vi "Testing_Original.vi"() -> ()   [LabVIEW 2021]
uses:
  Motion_Panel_State_Machine/Motion_Panel_State_Machine.lvclass
  C:/Program Files (x86)/Hyper State Machine Framework/SSW_Panel_Adaptive.lvlibp/Panel_Adaptive/Panel_Adaptive.lvclass
  C:/Program Files (x86)/Hyper State Machine Framework/SSW_Hyper_State_Machine.lvlibp/State_Machine_Class/Main_State_Machine/Hyper_State_Machine.lvclass
  DIO_Panel_State_Machine/DIO_Panel_State_Machine.lvclass
  Class 1/Panel1.lvclass
  C:/Program Files (x86)/Hyper State Machine Framework/SSW_Panel_Adaptive.lvlibp/Panel_Interface/Panel_Interface.lvclass
  Class 3/Panel3.lvclass
  Class 2/Panel2.lvclass
  C:/Program Files (x86)/Hyper State Machine Framework/SSW_Hyper_State_Machine.lvlibp/State_Machine_Class/State_Machine_Module.llb/Lock_Unlock.ctl
  C:/Program Files (x86)/Hyper State Machine Framework/SSW_Hyper_State_Machine.lvlibp/State_Machine_Class/State_Machine_Module.llb/State Machine.ctl
  C:/Program Files (x86)/Hyper State Machine Framework/SSW_Hyper_State_Machine.lvlibp
panel:
  out "Block_Chain":refnum<class "Hyper_State_Machine.lvclass">[](array[class])
  out "Commander":refnum<class "Hyper_State_Machine.lvclass">
  out "Exit":bool
  out "HPSMO4-20":refnum<class "Panel_Adaptive.lvclass">[](array[class])
  out "HPSMO2":refnum<class "Panel_Adaptive.lvclass">
  out "HSMO4-20":refnum<class "Hyper_State_Machine.lvclass">[](array[class])
  out "HSMO3":refnum<class "Hyper_State_Machine.lvclass">
  out "HPSMO3":refnum<class "DIO_Panel_State_Machine.lvclass">
  out "HSMO2":refnum<class "Hyper_State_Machine.lvclass">
  out "HSMO1":refnum<class "Hyper_State_Machine.lvclass">
  out "HPSMO1":refnum<class "Motion_Panel_State_Machine.lvclass">
  in  "Reset_State":bool
  in  "Reset_All":bool
  in  "Change_VI_All":bool
  in  "Panel Index":i32=1 min=1 max=20
  in  "Implementation":u16(ring)
  in  "Change_VI":bool
  out "Main_Active":bool
  in  "Main_Interval(s)":dbl=0.025 format="%.0p"
  in  "Option Button":bool=TRUE
  in  "Time Target (s)":dbl=30.0 format="%#_13g"
  in  "lock All":bool
  in  "Unlock":bool
  out "All_Values":variant[][](array[variant])
  out "error out":errorcluster
  in  "Exit":bool
  in  "Tab Control":T1(tab)
  in  "Swap3-4":bool
  in  "Swap1-4":bool
  in  "Swap2-3":bool
  in  "Swap1-2":bool
  out "Active 3":bool
  out "Active 2":bool
  out "Timing 3":dbl
  out "Timing 2":dbl
  out "Active 1":bool
  out "Timing 1":dbl
  out "Timing 20":dbl
  out "Active 20":bool
  out "Get_Current State_Sub Panel_1":string
  out "HSMO1_ID":u32 format="%08x"
  out "HSMO1 Running":bool
  in  "Request_Release":bool
  out "Command_Lock":bool
  out "Commander_State":string
  out "HSMO_Commander_ID":u32 format="%08x"
  out "Block Chain Message":string
  # "Local"
  # "Panel Method"
  # "State Method"
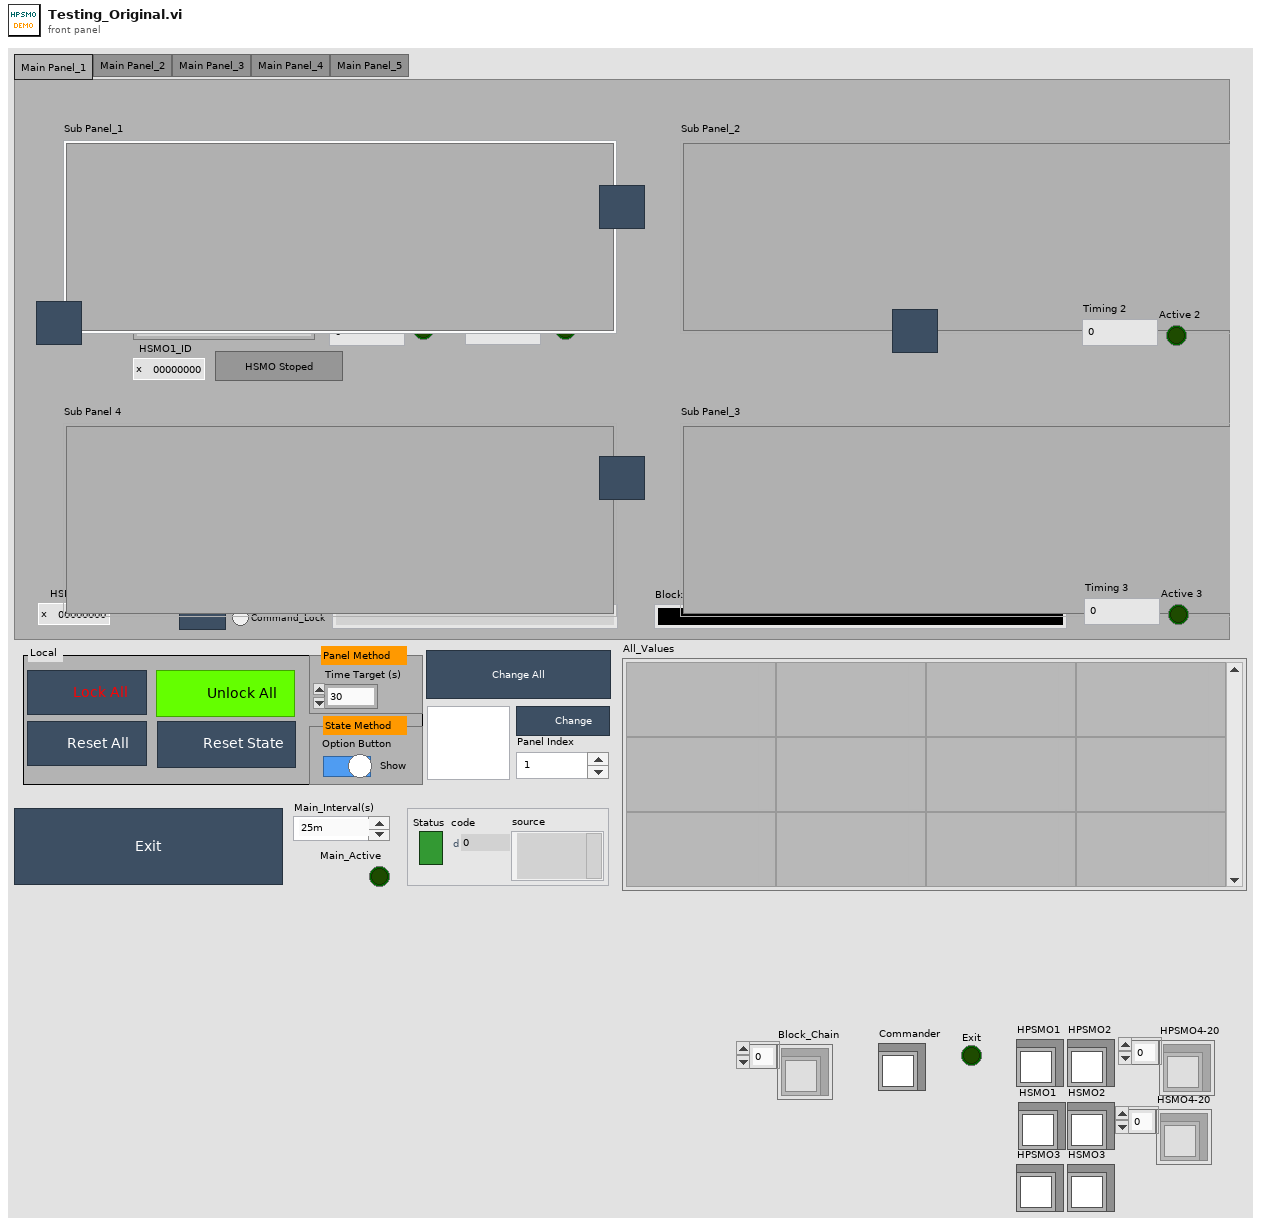
[diagram p1: front panel]
types:
  T1 = enum32{"Main Panel_1", "Main Panel_2", "Main Panel_3", "Main Panel_4", "Main Panel_5"}
  T2 = typedef "SSW_Hyper_State_Machine.lvlibp/State Machine.ctl" = cluster{"Command":string, "Data":variant}
  T3 = typedef "SSW_Hyper_State_Machine.lvlibp/Lock_Unlock.ctl" = cluster{"Action_Mode (Get)":enum16{"Set", "Get"}, "Action_Set (False)":bool, "State_In (Wait)":string}
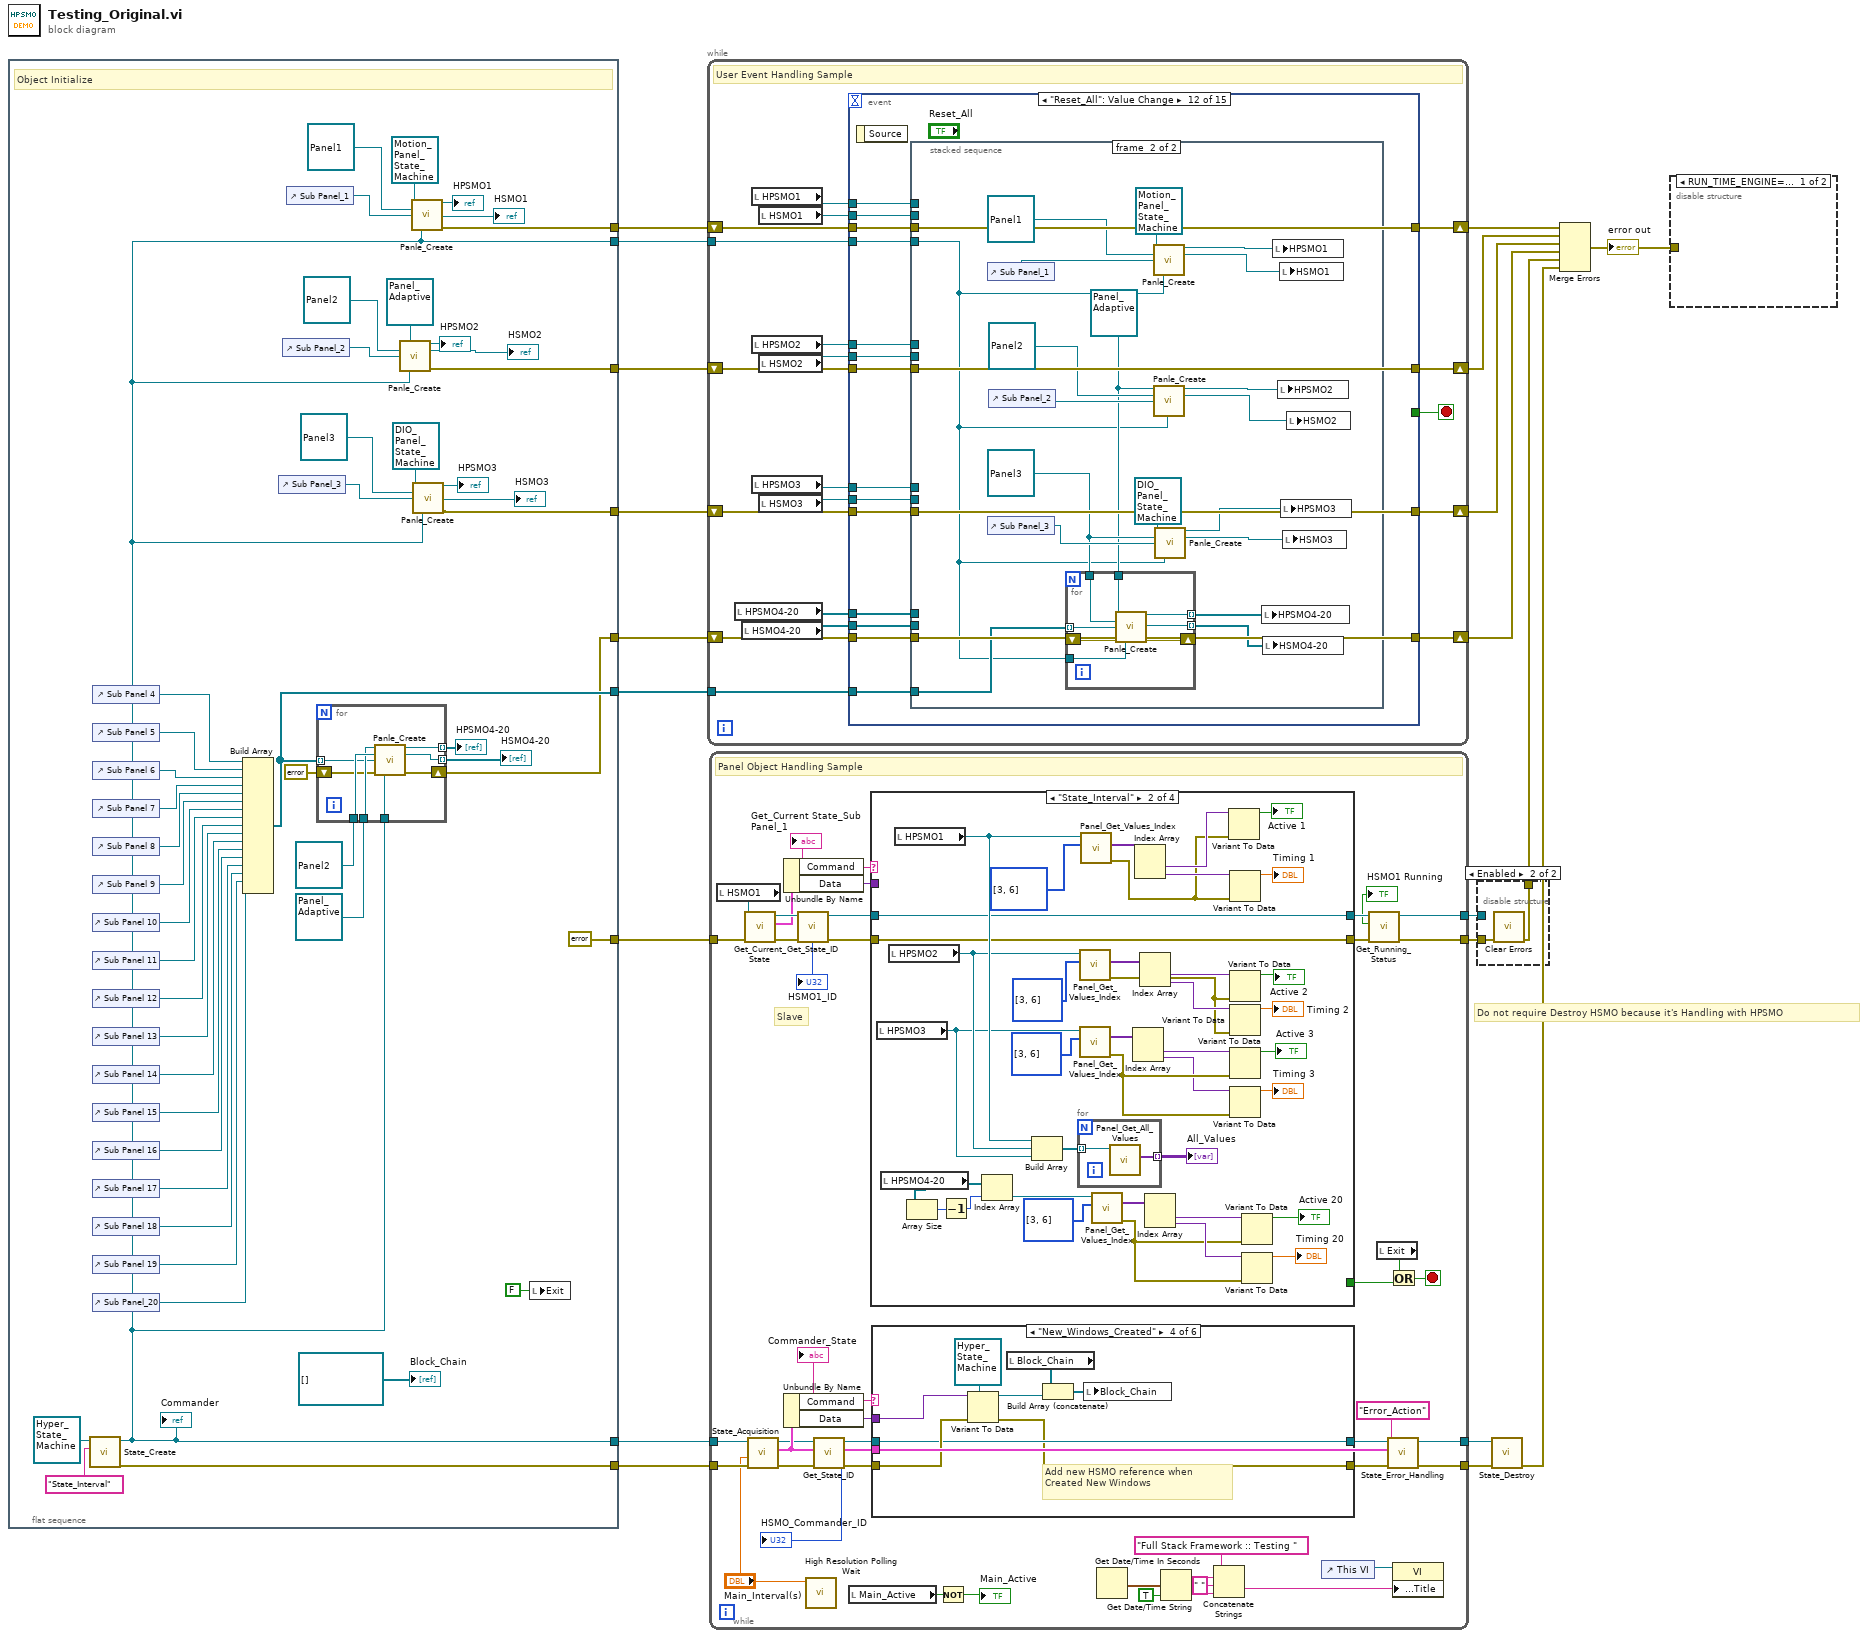
[diagram p0: block diagram]
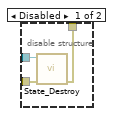
[diagram p2: hidden frame]
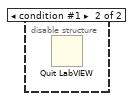
[diagram p3: hidden frame]
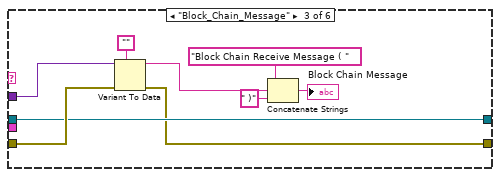
[diagram p6: hidden frame]
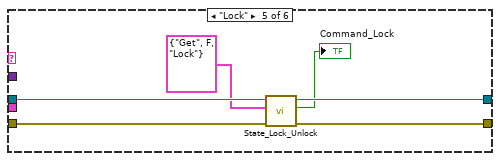
[diagram p7: hidden frame]
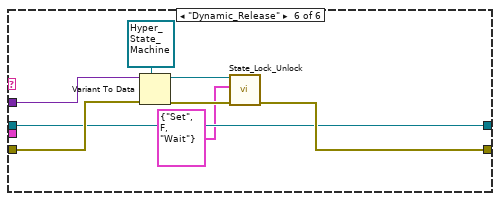
[diagram p8: hidden frame]
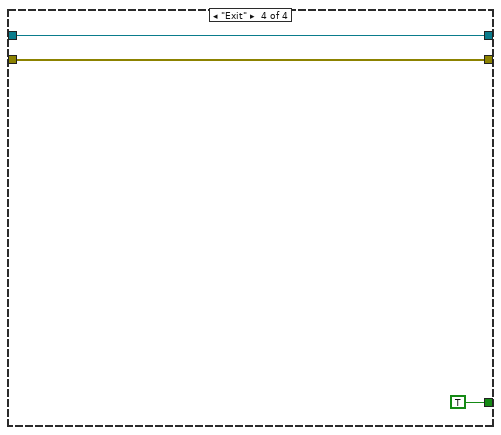
[diagram p11: hidden frame]
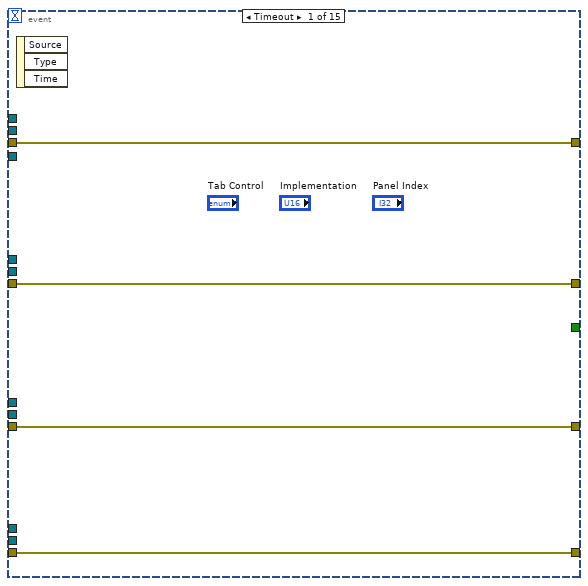
[diagram p12: hidden frame]
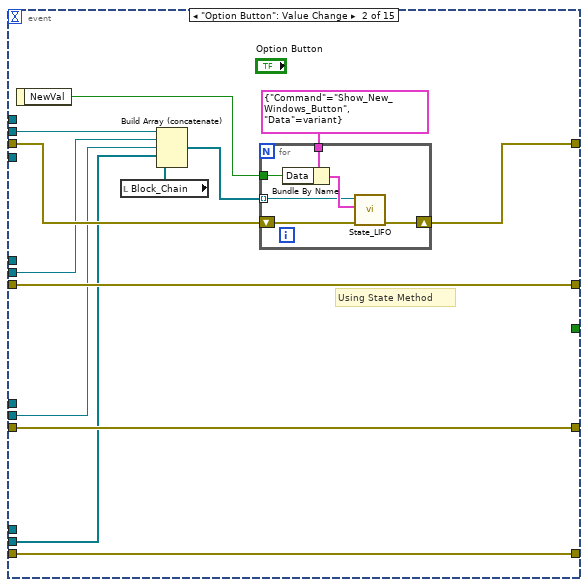
[diagram p13: hidden frame]
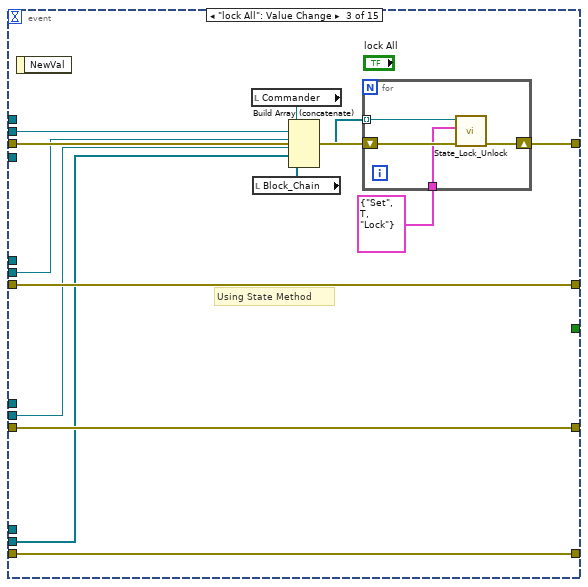
[diagram p14: hidden frame]
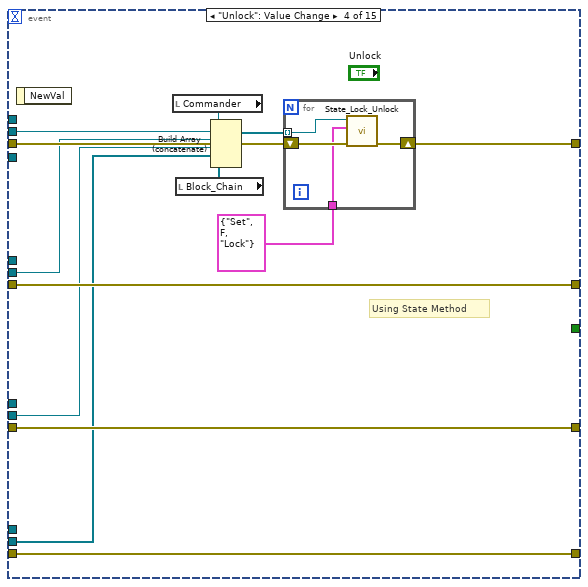
[diagram p15: hidden frame]
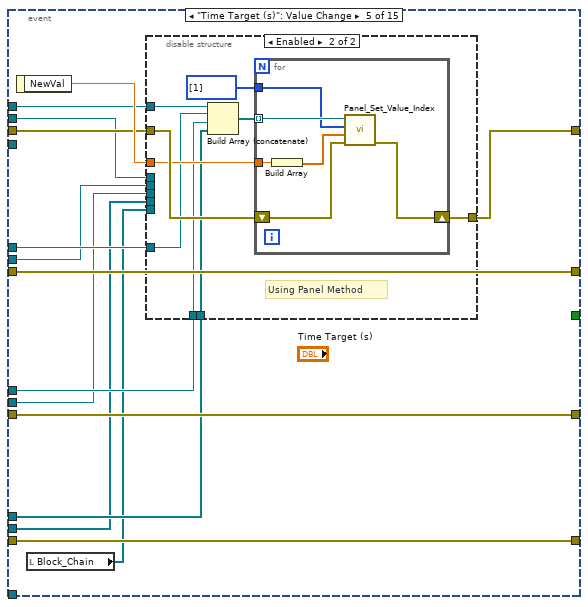
[diagram p16: hidden frame]
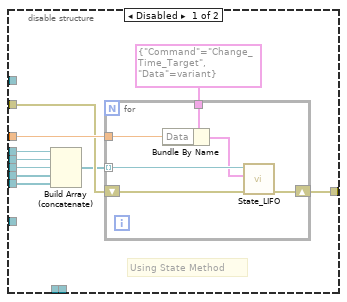
[diagram p17: hidden frame]
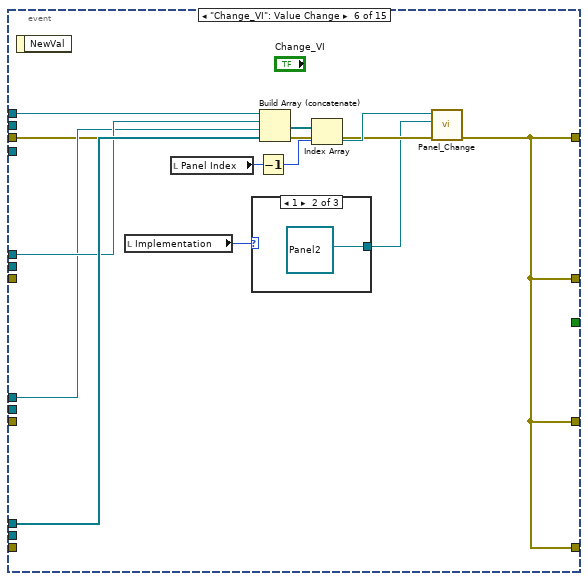
[diagram p18: hidden frame]
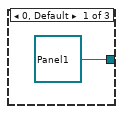
[diagram p19: hidden frame]
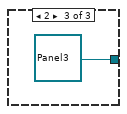
[diagram p20: hidden frame]
diagram:
  # "Do not require Destroy HSMO because it's Handling with HPSMO"
  n1 = flat-sequence {
    tunnel: [w41] -> w15
    tunnel: [w39] -> w9
    tunnel: [w38] -> w14
    tunnel: [w37] -> w13
    tunnel: [w32] -> w12
    tunnel: [errorcluster {"status"=FALSE, "code"=0, "source"=""} ("error in (no error)")] -> w4
    tunnel: [w21] -> w3
    tunnel: [w23] -> w2
    tunnel: [w21] -> w1
    frame #0 {
      # "Object Initialize"
      n2 = call-dynamic "State_Create.vi"("State_Interval_Name"="State_Interval", "State_Machine_Class in"=refnum<class "Hyper_State_Machine.lvclass"> refnum) -> ("error out"=w23:errorcluster, "State_Machine_Class out"=w21:refnum<class "Hyper_State_Machine.lvclass">)  [unwired: 7 in, 1 out]
      "Commander" <- w21
      n3 = control-ref of="Sub Panel 4"() -> (w64:refnum<vi>)
      n4 = control-ref of="Sub Panel 5"() -> (w63:refnum<vi>)
      n5 = control-ref of="Sub Panel 6"() -> (w62:refnum<vi>)
      n6 = control-ref of="Sub Panel 7"() -> (w61:refnum<vi>)
      n7 = control-ref of="Sub Panel 8"() -> (w60:refnum<vi>)
      n8 = control-ref of="Sub Panel 9"() -> (w59:refnum<vi>)
      n9 = control-ref of="Sub Panel 10"() -> (w58:refnum<vi>)
      n10 = control-ref of="Sub Panel 11"() -> (w57:refnum<vi>)
      n11 = control-ref of="Sub Panel 12"() -> (w56:refnum<vi>)
      n12 = control-ref of="Sub Panel 13"() -> (w55:refnum<vi>)
      n13 = control-ref of="Sub Panel 14"() -> (w54:refnum<vi>)
      n14 = control-ref of="Sub Panel 15"() -> (w53:refnum<vi>)
      n15 = control-ref of="Sub Panel 16"() -> (w52:refnum<vi>)
      n16 = control-ref of="Sub Panel 17"() -> (w51:refnum<vi>)
      n17 = control-ref of="Sub Panel 18"() -> (w50:refnum<vi>)
      n18 = control-ref of="Sub Panel 19"() -> (w49:refnum<vi>)
      n19 = control-ref of="Sub Panel_20"() -> (w47:refnum<vi>)
      n20 = Build Array(w64, w63, w62, w61, w60, w59, w58, w57, w56, w55, w54, w53, w52, w51, w50, w49, w47) -> (w41:refnum<vi>[])
      n21 = control-ref of="Sub Panel_3"() -> (w46:refnum<vi>)
      n22 = control-ref of="Sub Panel_2"() -> (w28:refnum<vi>)
      n23 = control-ref of="Sub Panel_1"() -> (w45:refnum<vi>)
      n24 = for {
        shift-right: [w73] -> w38
        shift-left: errorcluster {"status"=FALSE, "code"=0, "source"=""} ("error out") -> [w75]
        tunnel: w41 -> [w74] mode=indexing
        tunnel: [w72] -> w48 mode=indexing
        tunnel: refnum<class "Panel2.lvclass"> refnum ("Class 2.lvclass") -> [w77]
        tunnel: refnum<class "Panel_Adaptive.lvclass"> refnum ("SSW_Panel_Adaptive.lvlibp:Panel_Adaptive.lvclass") -> [w76]
        tunnel: [w71] -> w30 mode=indexing
        tunnel: w21 -> [w70]
        n25 = call-dynamic "Panle_Create.vi"("Hyper_Panel_State_Machine in"=w76, "Panel_Source"=w77, "Panel_Ref"=w74, "error in (no error)"=w75, "Parent_State"=w70) -> ("Hyper_Panel_State_Machine out"=w71:refnum<class "Panel_Adaptive.lvclass">, "This_State"=w72:refnum<class "Hyper_State_Machine.lvclass">, "error out"=w73:errorcluster)  [unwired: 8 in]
      }
      "HSMO4-20" <- w48
      "HPSMO4-20" <- w30
      n26 = call-dynamic "Panle_Create.vi"("Hyper_Panel_State_Machine in"=refnum<class "Panel_Adaptive.lvclass"> refnum ("SSW_Panel_Adaptive.lvlibp:Panel_Adaptive.lvclass"), "Panel_Source"=refnum<class "Panel2.lvclass"> refnum ("Class 2.lvclass"), "Panel_Ref"=w28, "Parent_State"=w21) -> ("Hyper_Panel_State_Machine out"=→"HPSMO2":refnum<class "Panel_Adaptive.lvclass">, "This_State"=→"HSMO2":refnum<class "Hyper_State_Machine.lvclass">, "error out"=w32:errorcluster)  [unwired: 9 in]
      n27 = call-dynamic "Panle_Create.vi"("Hyper_Panel_State_Machine in"=refnum<class "Motion_Panel_State_Machine.lvclass"> refnum ("Motion_Panel_State_Machine.lvclass"), "Panel_Source"=refnum<class "Panel1.lvclass"> refnum ("Class 1.lvclass"), "Panel_Ref"=w45, "Parent_State"=w21) -> ("Hyper_Panel_State_Machine out"=→"HPSMO1":refnum<class "Motion_Panel_State_Machine.lvclass">, "This_State"=→"HSMO1":refnum<class "Hyper_State_Machine.lvclass">, "error out"=w39:errorcluster)  [unwired: 9 in]
      n28 = call-dynamic "Panle_Create.vi"("Hyper_Panel_State_Machine in"=refnum<class "DIO_Panel_State_Machine.lvclass"> refnum ("DIO_Panel_State_Machine.lvclass"), "Panel_Source"=refnum<class "Panel3.lvclass"> refnum ("Class 3.lvclass"), "Panel_Ref"=w46, "Parent_State"=w21) -> ("Hyper_Panel_State_Machine out"=→"HPSMO3":refnum<class "DIO_Panel_State_Machine.lvclass">, "This_State"=→"HSMO3":refnum<class "Hyper_State_Machine.lvclass">, "error out"=w37:errorcluster)  [unwired: 9 in]
      n29 = local write "Exit"(FALSE ("Exit")) -> ()
      "Block_Chain" <- refnum<class "Hyper_State_Machine.lvclass">[] [] ("Block_Chain")
    }
  }
  n30 = while {
    tunnel: w15 -> [w91]
    shift-right: [w92] -> w16
    shift-left: w9 -> [w83]
    shift-right: [w95] -> w20
    shift-left: w12 -> [w81]
    shift-right: [w94] -> w19
    shift-left: w13 -> [w82]
    shift-right: [w93] -> w17
    shift-left: w14 -> [w80]
    tunnel: w1 -> [w78]
    stop <- w96 stop-if-true
    # "User Event Handling Sample"
    n31 = local read "HPSMO4-20"() -> (w87:refnum<class "Panel_Adaptive.lvclass">[])
    n32 = local read "HSMO4-20"() -> (w86:refnum<class "Hyper_State_Machine.lvclass">[])
    n33 = local read "HPSMO1"() -> (w90:refnum<class "Motion_Panel_State_Machine.lvclass">)
    n34 = local read "HPSMO2"() -> (w89:refnum<class "Panel_Adaptive.lvclass">)
    n35 = local read "HPSMO3"() -> (w85:refnum<class "DIO_Panel_State_Machine.lvclass">)
    n36 = local read "HSMO1"() -> (w79:refnum<class "Hyper_State_Machine.lvclass">)
    n37 = local read "HSMO2"() -> (w88:refnum<class "Hyper_State_Machine.lvclass">)
    n38 = local read "HSMO3"() -> (w84:refnum<class "Hyper_State_Machine.lvclass">)
    n39 = event shown="[11] \"Reset_All\": Value Change" {
      selector: _ -> [_ _ _ _ _ _ _ _ _ _ _ _ _ _ _]
      dyn-events: _ -> [_ _ _ _ _ _ _ _ _ _ _ _ _ _ _]
      timeout: _ -> [_ _ _ _ _ _ _ _ _ _ _ _ _ _ _]
      tunnel: [_ _ _ _ _ _ _ _ _ _ _ _ _ _ w365] -> w96
      tunnel: w83 -> [w98 w113 w131 w148 w166 w201 _ w240 w245 w261 w269 w281 w337 w350 w364]
      tunnel: [_ w112 w132 w149 w168 w209 w223 w239 w245 w258 w269 w281 w337 w347 w362] -> w92
      tunnel: w90 -> [_ _ _ _ w159 w204 w219 w233 _ w254 _ w282 _ _ w356]
      tunnel: w79 -> [_ w105 w125 w140 w158 _ _ _ _ _ _ w286 w333 w349 w352]
      tunnel: w88 -> [_ w104 w124 w141 w157 _ _ _ _ _ _ w285 w332 _ _]
      tunnel: w84 -> [_ w103 w123 w138 w156 _ _ _ _ _ _ w284 w331 _ _]
      tunnel: w89 -> [_ _ _ _ w160 w203 w218 w234 w243 _ _ w280 _ _ w355]
      tunnel: w85 -> [_ _ _ _ w161 w202 w217 _ w244 _ w266 w278 _ _ w354]
      tunnel: w81 -> [w99 w108 w128 w145 w163 _ _ w235 w250 w256 w270 w279 w336 _ w359]
      tunnel: [w98 _ _ _ _ _ _ _ _ _ _ _ _ _ _] -> _
      tunnel: [w99 w108 w128 w145 w163 w209 w223 w238 w248 w256 w270 w279 w336 _ w361] -> w95
      tunnel: [w100 w107 w127 w144 w164 w209 w223 w237 w247 w257 w265 w277 w335 _ w360] -> w94
      tunnel: w87 -> [_ _ _ _ w162 w205 w220 _ _ w253 w267 w276 _ _ w353]
      tunnel: w80 -> [w97 w106 w126 w143 w165 _ _ w236 w246 w260 w272 w275 w334 _ w358]
      tunnel: [w97 w106 w126 w143 w165 w209 w223 w236 w246 w259 w271 w275 w334 _ w357] -> w93
      tunnel: w86 -> [_ w102 w122 w142 w155 _ _ _ _ _ _ w283 w330 _ _]
      tunnel: w82 -> [w100 w107 w127 w144 w164 _ _ w237 w249 w257 w264 w277 w335 _ w363]
      tunnel: w91 -> [_ _ _ _ _ _ _ _ _ _ _ w274 _ _ _]
      tunnel: w78 -> [_ _ _ _ _ _ _ _ _ _ _ w273 _ _ _]
      event Timeout {
        n40 = event-data() -> ()  [unwired: 1 in, 3 out]
      }
      event "Option Button": Value Change {
        # "Using State Method"
        n41 = event-data() -> ("NewVal"=w111:bool)  [unwired: 1 in]
        n42 = local read "Block_Chain"() -> (w101:refnum<class "Hyper_State_Machine.lvclass">[])
        n43 = Build Array (concatenate)(w105, w104, w103, w102, w101) -> (w110:refnum<class "Hyper_State_Machine.lvclass">[])
        n44 = for {
          tunnel: w111 -> [w117]
          tunnel: w110 -> [w115] mode=indexing
          shift-right: [w118] -> w112
          shift-left: w113 -> [w119]
          tunnel: T2 {"Command"="Show_New_Windows_Button", "Data"=variant} ("State Machine") -> [w114]
          n45 = Bundle By Name(cluster=w114, "Data"=w117) -> (w116:T2)
          n46 = call-dynamic "State_LIFO.vi"("error in (no error)"=w119, "State Machine"=w116, "State_Machine_Class in"=w115) -> ("error out"=w118:errorcluster)  [unwired: 7 in, 1 out]
        }
      }
      event "lock All": Value Change {
        # "Using State Method"
        n47 = event-data() -> ()  [unwired: 1 in, 1 out]
        n48 = local read "Commander"() -> (w121:refnum<class "Hyper_State_Machine.lvclass">)
        n49 = local read "Block_Chain"() -> (w120:refnum<class "Hyper_State_Machine.lvclass">[])
        n50 = Build Array (concatenate)(w121, w125, w124, w123, w122, w120) -> (w130:refnum<class "Hyper_State_Machine.lvclass">[])
        n51 = for {
          tunnel: w130 -> [w134] mode=indexing
          shift-right: [w136] -> w132
          shift-left: w131 -> [w135]
          tunnel: T3 {"Action_Mode (Get)"=enum."Set", "Action_Set (False)"=TRUE, "State_In (Wait)"="Lock"} ("Parameter") -> [w133]
          n52 = call-dynamic "State_Lock_Unlock.vi"("error in (no error)"=w135, "Parameter"=w133, "State_Machine_Class in"=w134) -> ("error out"=w136:errorcluster)  [unwired: 6 in, 2 out]
        }
      }
      event "Unlock": Value Change {
        # "Using State Method"
        n53 = event-data() -> ()  [unwired: 1 in, 1 out]
        n54 = local read "Commander"() -> (w139:refnum<class "Hyper_State_Machine.lvclass">)
        n55 = local read "Block_Chain"() -> (w137:refnum<class "Hyper_State_Machine.lvclass">[])
        n56 = Build Array (concatenate)(w139, w140, w141, w138, w142, w137) -> (w147:refnum<class "Hyper_State_Machine.lvclass">[])
        n57 = for {
          tunnel: w147 -> [w152] mode=indexing
          shift-right: [w153] -> w149
          shift-left: w148 -> [w151]
          tunnel: T3 {"Action_Mode (Get)"=enum."Set", "Action_Set (False)"=FALSE, "State_In (Wait)"="Lock"} ("Parameter") -> [w150]
          n58 = call-dynamic "State_Lock_Unlock.vi"("error in (no error)"=w151, "Parameter"=w150, "State_Machine_Class in"=w152) -> ("error out"=w153:errorcluster)  [unwired: 6 in, 2 out]
        }
      }
      event "Time Target (s)": Value Change {
        n59 = event-data() -> ("NewVal"=w167:dbl)  [unwired: 1 in]
        n60 = local read "Block_Chain"() -> (w154:refnum<class "Hyper_State_Machine.lvclass">[])
        n61 = disable-structure shown="Enabled" {
          disable-tunnel: w158 -> [w177 _]
          disable-tunnel: [w176 w190] -> w168
          disable-tunnel: w167 -> [w178 w191]
          disable-tunnel: w159 -> [_ w193]
          disable-tunnel: w166 -> [w175 w192]
          disable-tunnel: w160 -> [_ w188]
          disable-tunnel: w161 -> [_ w187]
          disable-tunnel: w157 -> [w173 _]
          disable-tunnel: w156 -> [w172 _]
          disable-tunnel: w162 -> [_ w185]
          disable-tunnel: w155 -> [w170 _]
          disable-tunnel: w154 -> [w169 _]
          frame Disabled {
            # "Using State Method"
            n62 = Build Array (concatenate)(w177, w173, w172, w170, w169) -> (w174:refnum<class "Hyper_State_Machine.lvclass">[])
            n63 = for {
              tunnel: w178 -> [w184]
              tunnel: w174 -> [w183] mode=indexing
              shift-right: [w182] -> w176
              shift-left: w175 -> [w180]
              tunnel: T2 {"Command"="Change_Time_Target", "Data"=variant} ("State Machine") -> [w179]
              n64 = Bundle By Name(cluster=w179, "Data"=w184) -> (w181:T2)
              n65 = call-dynamic "State_LIFO.vi"("error in (no error)"=w180, "State Machine"=w181, "State_Machine_Class in"=w183) -> ("error out"=w182:errorcluster)  [unwired: 7 in, 1 out]
            }
          }
          frame Enabled {
            # "Using Panel Method"
            n66 = Build Array (concatenate)(w193, w188, w187, w185) -> (w189:refnum<class "Panel_Adaptive.lvclass">[])
            n67 = for {
              tunnel: w189 -> [w198] mode=indexing
              tunnel: w191 -> [w199]
              shift-right: [w194] -> w190
              shift-left: w192 -> [w195]
              tunnel: i32[] [1] ("Control_Indexes(Tabbing Order)") -> [w197]
              n68 = Build Array(w199) -> (w196:dbl[])
              n69 = call-dynamic "Panel_Set_Value_Index.vi"("error in (no error)"=w195, "Data_Values"=w196, "Control_Indexes(Tabbing Order)"=w197, "Hyper_Panel_State_Machine in"=w198) -> ("error out"=w194:errorcluster)  [unwired: 6 in, 1 out]
            }
          }
        }
      }
      event "Change_VI": Value Change {
        n70 = event-data() -> ()  [unwired: 1 in, 1 out]
        n71 = local read "Implementation"() -> (w206:u16)
        n72 = local read "Panel Index"() -> (w208:i32)
        n73 = case shown="1" w206 {
          tunnel: [refnum<class "Panel1.lvclass"> refnum ("Class 1.lvclass") refnum<class "Panel2.lvclass"> refnum ("Class 2.lvclass") refnum<class "Panel3.lvclass"> refnum ("Class 3.lvclass")] -> w200
          frame 0, Default {
          }
          frame 1 {
          }
          frame 2 {
          }
        }
        n74 = Decrement(x=w208) -> (x-1=w210:i32)
        n75 = Build Array (concatenate)(w204, w203, w202, w205) -> (w211:refnum<class "Panel_Adaptive.lvclass">[])
        n76 = Index Array(array=w211, index=w210) -> (element=w207:refnum<class "Panel_Adaptive.lvclass">)
        n77 = call-dynamic "Panel_Change.vi"("error in (no error)"=w201, "Panel_Source"=w200, "Hyper_Panel_State_Machine in"=w207) -> ("error out"=w209:errorcluster)  [unwired: 7 in, 1 out]
      }
      event "Change_VI_All": Value Change {
        n78 = event-data() -> ()  [unwired: 1 in, 1 out]
        n79 = local read "Implementation"() -> (w221:u16)
        n80 = Build Array (concatenate)(w219, w218, w217, w220) -> (w222:refnum<class "Panel_Adaptive.lvclass">[])
        n81 = case shown="0, Default" w221 {
          tunnel: [refnum<class "Panel1.lvclass"> refnum ("Class 1.lvclass") refnum<class "Panel2.lvclass"> refnum ("Class 2.lvclass") refnum<class "Panel3.lvclass"> refnum ("Class 3.lvclass")] -> w216
          frame 0, Default {
          }
          frame 1 {
          }
          frame 2 {
          }
        }
        n82 = for {
          tunnel: w222 -> [w226] mode=indexing
          tunnel: w216 -> [w225]
          shift-right: [w227] -> w223
          shift-left: errorcluster {"status"=FALSE, "code"=0, "source"=""} ("error out") -> [w224]
          n83 = call-dynamic "Panel_Change.vi"("error in (no error)"=w224, "Panel_Source"=w225, "Hyper_Panel_State_Machine in"=w226) -> ("error out"=w227:errorcluster)  [unwired: 7 in, 1 out]
        }
      }
      event "Swap1-2": Value Change {
        n84 = event-data() -> ()  [unwired: 1 in, 1 out]
        n85 = call-dynamic "Panel_Change.vi"("error in (no error)"=w240, "Interface_VI"=refnum<class "Panel2.lvclass"> refnum ("Class 2.lvclass"), "Hyper_Panel_State_Machine in"=w233) -> ("error out"=w239:errorcluster)  [unwired: 7 in, 1 out]
        n86 = call-dynamic "Panel_Change.vi"("error in (no error)"=w235, "Panel_Source"=refnum<class "Panel1.lvclass"> refnum ("Class 1.lvclass"), "Hyper_Panel_State_Machine in"=w234) -> ("error out"=w238:errorcluster)  [unwired: 7 in, 1 out]
      }
      event "Swap2-3": Value Change {
        n87 = event-data() -> ()  [unwired: 1 in, 1 out]
        n88 = call-dynamic "Panel_Change.vi"("error in (no error)"=w250, "Panel_Source"=refnum<class "Panel3.lvclass"> refnum ("Class 3.lvclass"), "Hyper_Panel_State_Machine in"=w243) -> ("error out"=w248:errorcluster)  [unwired: 7 in, 1 out]
        n89 = call-dynamic "Panel_Change.vi"("error in (no error)"=w249, "Interface_VI"=refnum<class "Panel2.lvclass"> refnum ("Class 2.lvclass"), "Hyper_Panel_State_Machine in"=w244) -> ("error out"=w247:errorcluster)  [unwired: 7 in, 1 out]
      }
      event "Swap1-4": Value Change {
        n90 = event-data() -> ()  [unwired: 1 in, 1 out]
        n91 = Index Array(array=w253) -> (element=w255:refnum<class "Panel_Adaptive.lvclass">)  [unwired: 1 in]
        n92 = call-dynamic "Panel_Change.vi"("error in (no error)"=w261, "Interface_VI"=refnum<class "Panel3.lvclass"> refnum ("Class 3.lvclass"), "Hyper_Panel_State_Machine in"=w254) -> ("error out"=w258:errorcluster)  [unwired: 7 in, 1 out]
        n93 = call-dynamic "Panel_Change.vi"("error in (no error)"=w260, "Panel_Source"=refnum<class "Panel1.lvclass"> refnum ("Class 1.lvclass"), "Hyper_Panel_State_Machine in"=w255) -> ("error out"=w259:errorcluster)  [unwired: 7 in, 1 out]
      }
      event "Swap3-4": Value Change {
        n94 = event-data() -> ()  [unwired: 1 in, 1 out]
        n95 = Index Array(array=w267) -> (element=w268:refnum<class "Panel_Adaptive.lvclass">)  [unwired: 1 in]
        n96 = call-dynamic "Panel_Change.vi"("error in (no error)"=w264, "Interface_VI"=refnum<class "Panel2.lvclass"> refnum ("Class 2.lvclass"), "Hyper_Panel_State_Machine in"=w266) -> ("error out"=w265:errorcluster)  [unwired: 7 in, 1 out]
        n97 = call-dynamic "Panel_Change.vi"("error in (no error)"=w272, "Panel_Source"=refnum<class "Panel3.lvclass"> refnum ("Class 3.lvclass"), "Hyper_Panel_State_Machine in"=w268) -> ("error out"=w271:errorcluster)  [unwired: 7 in, 1 out]
      }
      event "Reset_All": Value Change {
        n98 = event-data() -> ()  [unwired: 1 in, 1 out]
        n99 = stacked-sequence {
          tunnel: w286 -> [_ _]
          tunnel: w285 -> [_ _]
          tunnel: w284 -> [_ _]
          tunnel: w283 -> [_ _]
          tunnel: w282 -> [w296 _]
          tunnel: w281 -> [w295 _]
          tunnel: w280 -> [w294 _]
          tunnel: w279 -> [w293 _]
          tunnel: w278 -> [w292 _]
          tunnel: w277 -> [w291 _]
          tunnel: w276 -> [w290 _]
          tunnel: w275 -> [w289 _]
          tunnel: w274 -> [_ w313]
          tunnel: w273 -> [_ w302]
          frame #0 {
            # "Waiting Decision to Merage HPSMO and New HSMO (New Windows)"
            n100 = for {
              tunnel: w290 -> [w301] mode=indexing
              shift-right: [w299] -> _
              shift-left: w289 -> [w300]
              n101 = call-dynamic "Panel_Destroy.vi"("error in (no error)"=w300, "Hyper_Panel_State_Machine in"=w301) -> ("error out"=w299:errorcluster)  [unwired: 9 in]
            }
            n102 = call-dynamic "Panel_Destroy.vi"("error in (no error)"=w295, "Hyper_Panel_State_Machine in"=w296) -> ()  [unwired: 9 in, 1 out]
            n103 = call-dynamic "Panel_Destroy.vi"("error in (no error)"=w293, "Hyper_Panel_State_Machine in"=w294) -> ()  [unwired: 9 in, 1 out]
            n104 = call-dynamic "Panel_Destroy.vi"("error in (no error)"=w291, "Hyper_Panel_State_Machine in"=w292) -> ()  [unwired: 9 in, 1 out]
            n105 = local read "Block_Chain"() -> (w288:refnum<class "Hyper_State_Machine.lvclass">[])
            n106 = for {
              tunnel: w288 -> [w298] mode=indexing
              tunnel: [refnum<class "Hyper_State_Machine.lvclass">[] [] ("Block_Chain")] -> w287
              n107 = call-dynamic "State_Destroy.vi"("State_Machine_Class in"=w298) -> ()  [unwired: 10 in, 1 out]
            }
            n108 = local write "Block_Chain"(w287) -> ()
          }
          frame #1 {
            w303 = refnum<class "Panel_Adaptive.lvclass"> refnum ("SSW_Panel_Adaptive.lvlibp:Panel_Adaptive.lvclass")
            w314 = refnum<class "Panel3.lvclass"> refnum ("Class 3.lvclass")
            n109 = control-ref of="Sub Panel_1"() -> (w317:refnum<vi>)
            n110 = control-ref of="Sub Panel_3"() -> (w315:refnum<vi>)
            n111 = control-ref of="Sub Panel_2"() -> (w316:refnum<vi>)
            n112 = for {
              tunnel: w303 -> [w328]
              tunnel: [w327] -> w305 mode=indexing
              shift-right: [w325] -> _
              shift-left: _ -> [w326]
              tunnel: w313 -> [w323] mode=indexing
              tunnel: [w324] -> w304 mode=indexing
              tunnel: w314 -> [w322]
              tunnel: w302 -> [w321]
              n113 = call-dynamic "Panle_Create.vi"("Hyper_Panel_State_Machine in"=w328, "Panel_Source"=w322, "Panel_Ref"=w323, "error in (no error)"=w326, "Parent_State"=w321) -> ("Hyper_Panel_State_Machine out"=w327:refnum<class "Panel_Adaptive.lvclass">, "This_State"=w324:refnum<class "Hyper_State_Machine.lvclass">, "error out"=w325:errorcluster)  [unwired: 8 in]
            }
            n114 = call-dynamic "Panle_Create.vi"("Hyper_Panel_State_Machine in"=refnum<class "Motion_Panel_State_Machine.lvclass"> refnum ("Motion_Panel_State_Machine.lvclass"), "Panel_Source"=refnum<class "Panel1.lvclass"> refnum ("Class 1.lvclass"), "Panel_Ref"=w317, "Parent_State"=w302) -> ("Hyper_Panel_State_Machine out"=w311:refnum<class "Motion_Panel_State_Machine.lvclass">, "This_State"=w310:refnum<class "Hyper_State_Machine.lvclass">)  [unwired: 9 in, 1 out]
            n115 = call-dynamic "Panle_Create.vi"("Hyper_Panel_State_Machine in"=w303, "Panel_Source"=refnum<class "Panel2.lvclass"> refnum ("Class 2.lvclass"), "Panel_Ref"=w316, "Parent_State"=w302) -> ("Hyper_Panel_State_Machine out"=w309:refnum<class "Panel_Adaptive.lvclass">, "This_State"=w308:refnum<class "Hyper_State_Machine.lvclass">)  [unwired: 9 in, 1 out]
            n116 = call-dynamic "Panle_Create.vi"("Hyper_Panel_State_Machine in"=refnum<class "DIO_Panel_State_Machine.lvclass"> refnum ("DIO_Panel_State_Machine.lvclass"), "Panel_Source"=w314, "Panel_Ref"=w315, "Parent_State"=w302) -> ("Hyper_Panel_State_Machine out"=w307:refnum<class "DIO_Panel_State_Machine.lvclass">, "This_State"=w306:refnum<class "Hyper_State_Machine.lvclass">)  [unwired: 9 in, 1 out]
            n117 = local write "HPSMO4-20"(w305) -> ()
            n118 = local write "HSMO4-20"(w304) -> ()
            n119 = local write "HPSMO1"(w311) -> ()
            n120 = local write "HPSMO2"(w309) -> ()
            n121 = local write "HSMO1"(w310) -> ()
            n122 = local write "HPSMO3"(w307) -> ()
            n123 = local write "HSMO3"(w306) -> ()
            n124 = local write "HSMO2"(w308) -> ()
          }
        }
      }
      event "Reset_State": Value Change {
        n125 = event-data() -> ()  [unwired: 1 in, 1 out]
        n126 = local read "Block_Chain"() -> (w329:refnum<class "Hyper_State_Machine.lvclass">[])
        n127 = Build Array (concatenate)(w333, w332, w331, w330, w329) -> (w339:refnum<class "Hyper_State_Machine.lvclass">[])
        n128 = for {
          tunnel: w339 -> [w343] mode=indexing
          tunnel: T2 {"Command"="State_Init", "Data"=variant} ("State Machine") -> [w340]
          n129 = call-dynamic "State_Release.vi"("State_Machine_Class in"=w343) -> ("error out"=w341:errorcluster, "State_Machine_Class out"=w342:refnum<class "Hyper_State_Machine.lvclass">)  [unwired: 9 in]
          n130 = call-dynamic "State_LIFO.vi"("error in (no error)"=w341, "State Machine"=w340, "State_Machine_Class in"=w342) -> ()  [unwired: 7 in, 2 out]
        }
      }
      event "Request_Release": Value Change {
        n131 = event-data() -> ()  [unwired: 1 in, 1 out]
        n132 = local read "Commander"() -> (w344:refnum<class "Hyper_State_Machine.lvclass">)
        n133 = call-dynamic "State_Lock_Unlock.vi"("error in (no error)"=w350, "Parameter"=T3 {"Action_Mode (Get)"=enum."Set", "Action_Set (False)"=TRUE, "State_In (Wait)"="Lock"}, "State_Machine_Class in"=w344) -> ("error out"=w348:errorcluster)  [unwired: 6 in, 2 out]
        n134 = Bundle By Name(cluster=T2 {"Command"="Member_Release", "Data"=variant} ("State Machine"), "Data"=w344) -> (w345:T2)
        n135 = call-dynamic "State_LIFO.vi"("error in (no error)"=w348, "State Machine"=w345, "State_Machine_Class in"=w349) -> ("error out"=w347:errorcluster)  [unwired: 7 in, 1 out]
      }
      event "Exit": Value Change {
        n136 = event-data() -> ()  [unwired: 1 in, 1 out]
        n137 = Two Button Dialog(message="Exit Confirm") -> (T button?=w365:bool)  [unwired: 2 in]
        "Exit" <- w365
        n138 = case shown="True" w365 {
          tunnel: w364 -> [w370 w372]
          tunnel: w355 -> [_ w375]
          tunnel: w356 -> [_ w383]
          tunnel: w354 -> [_ w382]
          tunnel: w363 -> [w368 w381]
          tunnel: [w370 w380] -> w362
          tunnel: [w369 w373] -> w361
          tunnel: [w368 w379] -> w360
          tunnel: w359 -> [w369 w374]
          tunnel: w353 -> [_ w378]
          tunnel: w358 -> [w367 w377]
          tunnel: [w367 w376] -> w357
          tunnel: w352 -> [_ _]
          frame False {
          }
          frame True {
            n139 = local read "Block_Chain"() -> (w371:refnum<class "Hyper_State_Machine.lvclass">[])
            n140 = for {
              tunnel: w378 -> [w387] mode=indexing
              shift-right: [w385] -> w376
              shift-left: w377 -> [w386]
              n141 = call-dynamic "Panel_Destroy.vi"("error in (no error)"=w386, "Hyper_Panel_State_Machine in"=w387) -> ("error out"=w385:errorcluster)  [unwired: 9 in]
            }
            n142 = for {
              tunnel: w371 -> [w384] mode=indexing
              n143 = call-dynamic "State_Destroy.vi"("State_Machine_Class in"=w384) -> ()  [unwired: 10 in, 1 out]
            }
            n144 = call-dynamic "Panel_Destroy.vi"("error in (no error)"=w372, "Hyper_Panel_State_Machine in"=w383) -> ("error out"=w380:errorcluster)  [unwired: 9 in]
            n145 = call-dynamic "Panel_Destroy.vi"("error in (no error)"=w374, "Hyper_Panel_State_Machine in"=w375) -> ("error out"=w373:errorcluster)  [unwired: 9 in]
            n146 = call-dynamic "Panel_Destroy.vi"("error in (no error)"=w381, "Hyper_Panel_State_Machine in"=w382) -> ("error out"=w379:errorcluster)  [unwired: 9 in]
          }
        }
      }
    }
  }
  n147 = while {
    tunnel: [w409] -> w11
    tunnel: [w408] -> w8
    tunnel: w3 -> [w404]
    tunnel: w2 -> [w403]
    tunnel: [w396] -> w7
    tunnel: [w395] -> w6
    tunnel: w4 -> [w393]
    stop <- w418 stop-if-true
    # "Slave"
    # "Panel Object Handling Sample"
    n148 = local read "HSMO1"() -> (w420:refnum<class "Hyper_State_Machine.lvclass">)
    n149 = call-dynamic "Get_Current_State.vi"("error in (no error)"=w393, "Hyper_State_Machine in"=w420) -> ("error out"=w414:errorcluster, "Current_State"=w407:T2, "Hyper_State_Machine out"=w415:refnum<class "Hyper_State_Machine.lvclass">)  [unwired: 7 in]
    n150 = call-dynamic "State_Acquisition.vi"("error in (no error)"=w403, "State_Interval_Time(s)"="Main_Interval(s)", "Main_Machine_State_Class in"=w404) -> ("error out"=w391:errorcluster, "State"=w400:T2, "Main_Machine_State_Class out"=w392:refnum<class "Hyper_State_Machine.lvclass">)  [unwired: 2 in, 4 out]
    n151 = Unbundle By Name(w407) -> ("Command"=w405:string, "Data"=w406:variant)
    "Get_Current State_Sub Panel_1" <- w405
    n152 = Unbundle By Name(w400) -> ("Command"=w401:string, "Data"=w394:variant)
    "Commander_State" <- w401
    n153 = call-dynamic "Get_State_ID.vi"("error in (no error)"=w414, "Hyper_State_Machine in"=w415) -> ("error out"=w417:errorcluster, "State_ID"=→"HSMO1_ID":u32, "Hyper_State_Machine out"=w419:refnum<class "Hyper_State_Machine.lvclass">)  [unwired: 7 in]
    n154 = call <vilib>:"High Resolution Polling Wait.vi"("seconds to wait"="Main_Interval(s)") -> ()  [unwired: 10 in, 1 out]
    n155 = call-dynamic "Get_State_ID.vi"("error in (no error)"=w391, "Hyper_State_Machine in"=w392) -> ("error out"=w389:errorcluster, "State_ID"=→"HSMO_Commander_ID":u32, "Hyper_State_Machine out"=w390:refnum<class "Hyper_State_Machine.lvclass">)  [unwired: 7 in]
    n156 = local read "Main_Active"() -> (w431:bool)
    n157 = case shown="\"State_Interval\"" w405 {
      tunnel: w417 -> [w467 w472 w510 w512]
      tunnel: w419 -> [w468 w473 w511 w513]
      tunnel: [w468 w473 w511 w513] -> w413
      tunnel: [w467 w472 w510 w512] -> w412
      tunnel: [_ _ _ TRUE] -> w421
      tunnel: w406 -> [_ _ _ _]
      frame "Idle", Default {
      }
      frame "State_Interval" {
        n158 = local read "HPSMO3"() -> (w474:refnum<class "DIO_Panel_State_Machine.lvclass">)
        n159 = local read "HPSMO4-20"() -> (w471:refnum<class "Panel_Adaptive.lvclass">[])
        n160 = local read "HPSMO2"() -> (w475:refnum<class "Panel_Adaptive.lvclass">)
        n161 = local read "HPSMO1"() -> (w476:refnum<class "Motion_Panel_State_Machine.lvclass">)
        n162 = Array Size(array=w471) -> (size(s)=w470:i32)
        n163 = Decrement(x=w470) -> (x-1=w469:i32)
        n164 = Index Array(array=w471, index=w469) -> (element=w479:refnum<class "Panel_Adaptive.lvclass">)
        n165 = Build Array(w476, w475, w474) -> (w489:refnum<class "Panel_Adaptive.lvclass">[])
        n166 = for {
          tunnel: w489 -> [w509] mode=indexing
          tunnel: [w508] -> w488 mode=indexing
          n167 = call-dynamic "Panel_Get_All_Values.vi"("Hyper_Panel_State_Machine in"=w509) -> ("All_Values"=w508:variant[])  [unwired: 8 in, 2 out]
        }
        "All_Values" <- w488
        n168 = call-dynamic "Panel_Get_Values_Index.vi"("Control_Indexes(Tabbing Order)"=i32[] [3, 6], "Hyper_Panel_State_Machine in"=w475) -> ("error out"=w485:errorcluster, "Data_Values"=w486:variant[])  [unwired: 7 in, 1 out]
        n169 = call-dynamic "Panel_Get_Values_Index.vi"("Control_Indexes(Tabbing Order)"=i32[] [3, 6], "Hyper_Panel_State_Machine in"=w474) -> ("error out"=w507:errorcluster, "Data_Values"=w498:variant[])  [unwired: 7 in, 1 out]
        n170 = call-dynamic "Panel_Get_Values_Index.vi"("Control_Indexes(Tabbing Order)"=i32[] [3, 6] ("control indexes"), "Hyper_Panel_State_Machine in"=w476) -> ("error out"=w490:errorcluster, "Data_Values"=w497:variant[])  [unwired: 7 in, 1 out]
        n171 = call-dynamic "Panel_Get_Values_Index.vi"("Control_Indexes(Tabbing Order)"=i32[] [3, 6], "Hyper_Panel_State_Machine in"=w479) -> ("error out"=w480:errorcluster, "Data_Values"=w483:variant[])  [unwired: 7 in, 1 out]
        n172 = Index Array(array=w498) -> (element #1=w504:variant, element #2=w502:variant)  [unwired: 2 in]
        n173 = Index Array(array=w497) -> (element #1=w493:variant, element #2=w495:variant)  [unwired: 2 in]
        n174 = Index Array(array=w486) -> (element #1=w503:variant, element #2=w501:variant)  [unwired: 2 in]
        n175 = Index Array(array=w483) -> (element #1=w481:variant, element #2=w482:variant)  [unwired: 2 in]
        n176 = Variant To Data(error in=w490, Variant=w493) -> (data=→"Active 1":bool)  [unwired: 1 in, 1 out]
        n177 = Variant To Data(error in=w490, Variant=w495) -> (data=→"Timing 1":dbl)  [unwired: 1 in, 1 out]
        n178 = Variant To Data(error in=w485, Variant=w503) -> (data=→"Active 2":bool)  [unwired: 1 in, 1 out]
        n179 = Variant To Data(error in=w485, Variant=w501) -> (data=→"Timing 2":dbl)  [unwired: 1 in, 1 out]
        n180 = Variant To Data(error in=w507, Variant=w504) -> (data=→"Active 3":bool)  [unwired: 1 in, 1 out]
        n181 = Variant To Data(error in=w507, Variant=w502) -> (data=→"Timing 3":dbl)  [unwired: 1 in, 1 out]
        n182 = Variant To Data(error in=w480, Variant=w481) -> (data=→"Active 20":bool)  [unwired: 1 in, 1 out]
        n183 = Variant To Data(error in=w480, Variant=w482) -> (data=→"Timing 20":dbl)  [unwired: 1 in, 1 out]
      }
      frame "Error_Action" {
      }
      frame "Exit" {
      }
    }
    n184 = case shown="\"New_Windows_Created\"" w401 {
      tunnel: w390 -> [w433 w435 w442 w450 w458 w460]
      tunnel: w389 -> [w432 w434 w443 w451 w457 w464]
      tunnel: w400 -> [_ _ _ _ _ _]
      tunnel: [w433 w435 w442 w450 w455 w460] -> w399
      tunnel: [w432 w434 w437 w449 w454 w461] -> w398
      tunnel: w394 -> [_ _ w444 w452 _ w466]
      frame "Idle", Default {
      }
      frame "State_Interval" {
      }
      frame "Block_Chain_Message" {
        n185 = Variant To Data(error in=w443, type="", Variant=w444) -> (data=w438:string, error out=w437:errorcluster)
        n186 = Concatenate Strings("Block Chain Receive Message ( " ("string"), w438, " )" ("string")) -> (→"Block Chain Message":string)
      }
      frame "New_Windows_Created" {
        # "Add new HSMO reference when\nCreated New Windows"
        n187 = Variant To Data(error in=w451, type=refnum<class "Hyper_State_Machine.lvclass"> refnum ("Hyper_State_Machine out"), Variant=w452) -> (data=w446:refnum<class "Hyper_State_Machine.lvclass">, error out=w449:errorcluster)
        n188 = local read "Block_Chain"() -> (w448:refnum<class "Hyper_State_Machine.lvclass">[])
        n189 = Build Array (concatenate)(w448, w446) -> (w447:refnum<class "Hyper_State_Machine.lvclass">[])
        n190 = local write "Block_Chain"(w447) -> ()
      }
      frame "Lock" {
        n191 = call-dynamic "State_Lock_Unlock.vi"("error in (no error)"=w457, "Parameter"=T3 {"Action_Mode (Get)"=enum."Get", "Action_Set (False)"=FALSE, "State_In (Wait)"="Lock"}, "State_Machine_Class in"=w458) -> ("error out"=w454:errorcluster, "Action_Get"=→"Command_Lock":bool, "State_Machine_Class out"=w455:refnum<class "Hyper_State_Machine.lvclass">)  [unwired: 6 in]
      }
      frame "Dynamic_Release" {
        n192 = Variant To Data(error in=w464, type=refnum<class "Hyper_State_Machine.lvclass"> refnum ("State_Machine_Class in"), Variant=w466) -> (data=w463:refnum<class "Hyper_State_Machine.lvclass">, error out=w462:errorcluster)
        n193 = call-dynamic "State_Lock_Unlock.vi"("error in (no error)"=w462, "Parameter"=T3 {"Action_Mode (Get)"=enum."Set", "Action_Set (False)"=FALSE, "State_In (Wait)"="Wait"}, "State_Machine_Class in"=w463) -> ("error out"=w461:errorcluster)  [unwired: 6 in, 2 out]
      }
    }
    n194 = Not(x=w431) -> (.not. x?=→"Main_Active":bool)
    n195 = Get Date/Time In Seconds() -> (seconds since 1Jan1904=w429:timestamp)
    n196 = Get Date/Time String(seconds (now)=w429, want seconds? (F)=TRUE) -> (date string=w427:string, time string=w423:string)  [unwired: 1 in]
    n197 = Concatenate Strings("Full Stack Framework :: Testing " ("string"), w427, " " ("string"), w423) -> (w425:string)
    n198 = control-ref of="This VI"() -> (w422:refnum<vi>)
    n199 = call-dynamic "Get_Running_Status.vi"("error in (no error)"=w412, "Hyper_State_Machine in"=w413) -> ("error out"=w408:errorcluster, "State_Running"=→"HSMO1 Running":bool, "Hyper_State_Machine out"=w409:refnum<class "Hyper_State_Machine.lvclass">)  [unwired: 7 in]
    n200 = local read "Exit"() -> (w410:bool)
    n201 = call-dynamic "State_Error_Handling.vi"("error in (no error)"=w398, "Reply_State_Name"="Error_Action", "Handling_State(State_Acquisition)"=w400, "State_Machine_Class in"=w399) -> ("error out"=w396:errorcluster, "State_Machine_Class out"=w395:refnum<class "Hyper_State_Machine.lvclass">)  [unwired: 6 in]
    n202 = Or(x=w410, y=w421) -> (x .or. y?=w418:bool)
    n203 = property class="VI"(reference=w422, "Front Panel.Title"=w425) -> ()  [unwired: 1 in, 2 out]
  }
  n204 = disable-structure shown="Enabled" {
    disable-tunnel: w8 -> [w517 w519]
    disable-tunnel: w11 -> [w516 _]
    disable-tunnel: [w515 w518] -> w10
    frame Disabled {
      n205 = call-dynamic "State_Destroy.vi"("error in (no error)"=w517, "State_Machine_Class in"=w516) -> ("error out"=w515:errorcluster)  [unwired: 9 in]
    }
    frame Enabled {
      n206 = call <vilib>:"Clear Errors.vi"("error in (no error)"=w519) -> ("error out"=w518:errorcluster)  [unwired: 5 in, 1 out]
    }
  }
  n207 = call-dynamic "State_Destroy.vi"("error in (no error)"=w7, "State_Machine_Class in"=w6) -> ("error out"=w5:errorcluster)  [unwired: 9 in]
  n208 = Merge Errors(w16, w20, w19, w17, w10, w5) -> (w18:errorcluster)
  "error out" <- w18
  n209 = disable-structure shown="RUN_TIME_ENGINE==False, Default" {
    disable-tunnel: w18 -> [_ _]
    frame condition #0 (active) {
    }
    frame condition #1 {
      n210 = Quit LabVIEW() -> ()  [unwired: 1 in]
    }
  }
